vi "SMS_to_mobile.vi"(1 "SMS address":string[](array[string])=["SMS to Mobile:enflo@froude.mech.surrey.ac.uk"], 2 "Subject":string="Comms check", 3 "Message":string) -> (5 "error out":errorcluster)   [LabVIEW 2010]
uses:
  Globals/Preference_global.vi
panel:
  in  "Case Constant\n(See Context Help)":bool
  out "Number of SMS's sent today":i32
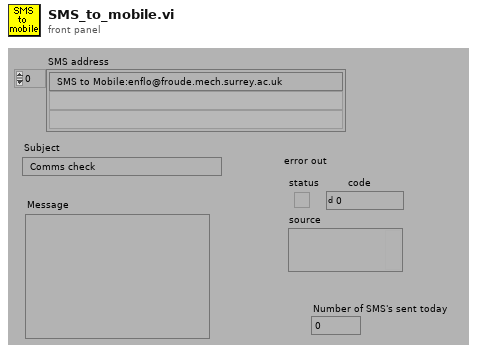
[diagram p1: front panel]
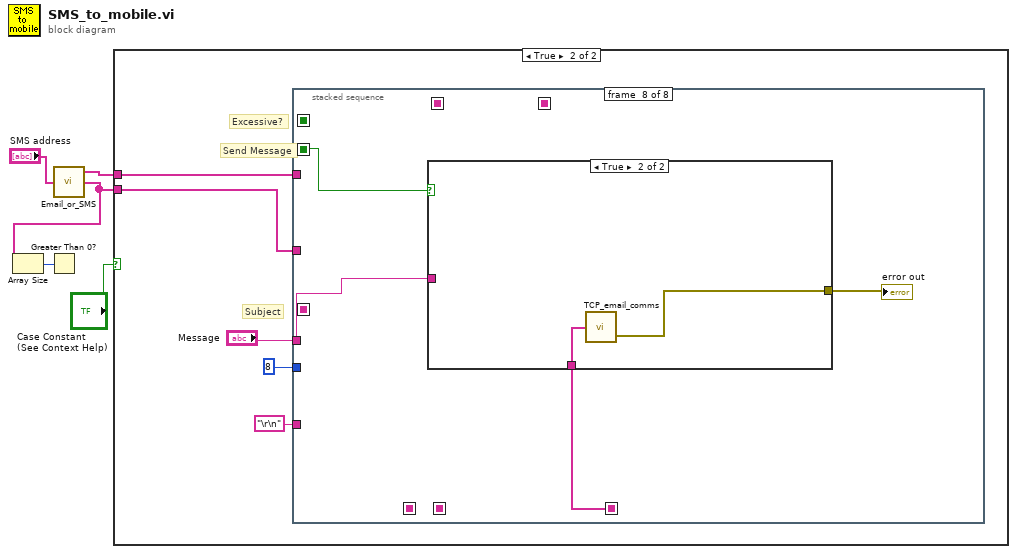
[diagram p0: block diagram]
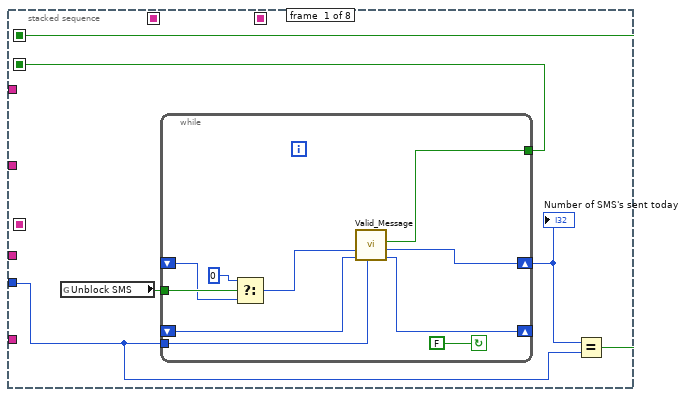
[diagram p3: hidden frame]
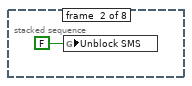
[diagram p4: hidden frame]
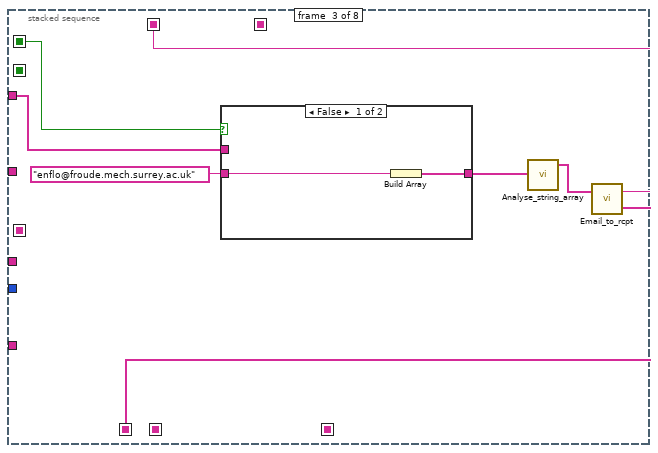
[diagram p5: hidden frame]
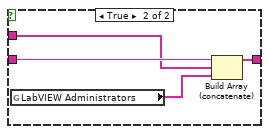
[diagram p6: hidden frame]
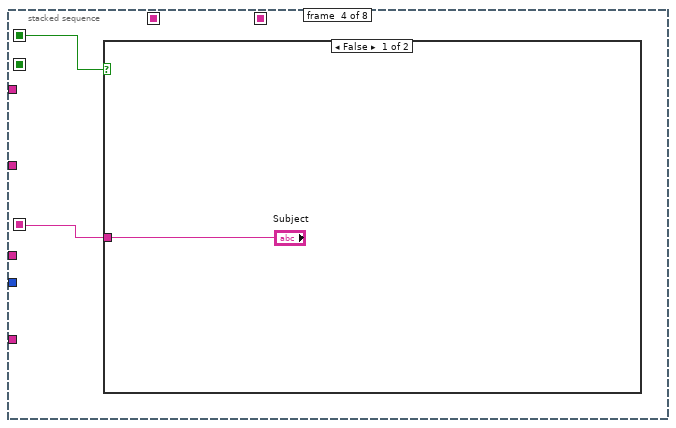
[diagram p7: hidden frame]
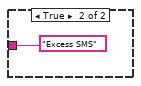
[diagram p8: hidden frame]
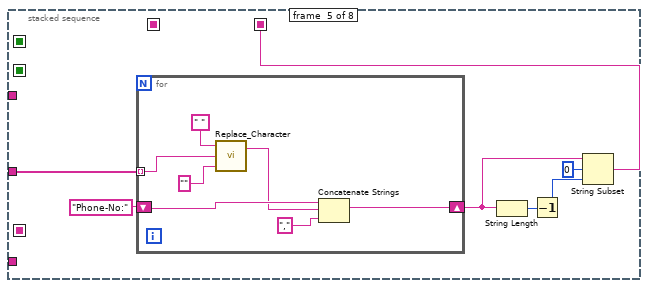
[diagram p9: hidden frame]
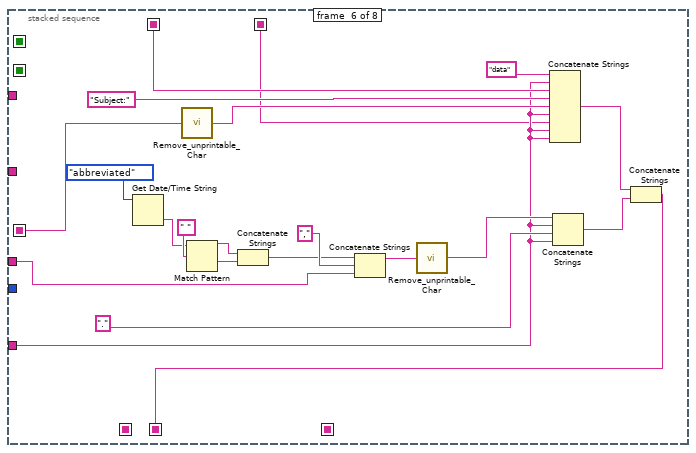
[diagram p10: hidden frame]
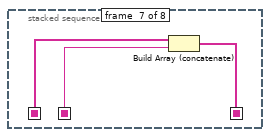
[diagram p11: hidden frame]
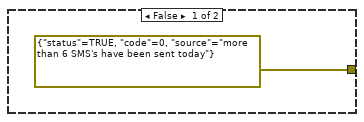
[diagram p12: hidden frame]
diagram:
  n1 = call "Email_or_SMS.vi"("Email address"="SMS address") -> ("Email"=w3:string[], "SMS to send"=w2:string[])  [unwired: 2 out]
  n2 = Array Size(array=w2) -> (size(s)=w4:i32)
  n3 = Greater Than 0?(x=w4) -> ()  [unwired: 1 out]
  n4 = case shown="True" "Case Constant\n(See Context Help)" {
    tunnel: w2 -> [_ w6]
    tunnel: w3 -> [_ w7]
    frame False {
    }
    frame True {
      # "Subject"
      # "Send Message"
      # "Excessive?"
      n5 = stacked-sequence {
        seq-local: [_ _ w28 _ _ _ _ _] -> [_ _ _ _ _ _ w80 _]
        seq-local: [_ _ w29 _ _ _ _ _] -> [_ _ _ _ _ w77 _ _]
        seq-local: [_ _ _ _ _ w73 _ _] -> [_ _ _ _ _ _ w81 _]
        seq-local: [_ _ _ _ _ _ w79 _] -> [_ _ _ _ _ _ _ w83]
        seq-local: [w14 _ _ _ _ _ _ _] -> [_ _ _ _ _ _ _ w84]
        seq-local: [w11 _ _ _ _ _ _ _] -> [_ _ w33 w40 _ _ _ _]
        seq-local: [_ _ _ w41 _ _ _ _] -> [_ _ _ _ _ w61 _ _]
        seq-local: [_ _ _ _ w44 _ _ _] -> [_ _ _ _ _ w58 _ _]
        tunnel: "\r\n" -> [_ _ _ _ _ w59 _ _]
        tunnel: w6 -> [_ _ _ _ w50 _ _ _]
        tunnel: 8 ("y") -> [w13 _ _ _ _ _ _ _]
        tunnel: "Message" -> [_ _ _ _ _ w60 _ w82]
        tunnel: w7 -> [_ _ w32 _ _ _ _ _]
        frame #0 {
          n6 = global read "Preference_global.vi" "Unblock SMS"() -> (w15:bool)
          n7 = while {
            tunnel: w15 -> [w20]
            tunnel: w13 -> [w22]
            tunnel: [w23] -> w14
            shift-left: _ -> [w19]
            shift-right: [w21] -> w12
            shift-left: _ -> [w25]
            shift-right: [w24] -> _
            stop <- FALSE continue-if-true
            n8 = Select(t=0, s=w20, f=w19) -> (s? t:f=w18:i32)
            n9 = call "Valid_Message.vi"("Max per day"=w22, "day of month in"=w25, "Number of requests today In"=w18) -> ("day of month out"=w24:i32, "Number of requests today Out"=w21:i32, "Send Message"=w23:bool)  [unwired: 2 in, 4 out]
          }
          "Number of SMS's sent today" <- w12
          n10 = Equal?(x=w12, y=w13) -> (x = y?=w11:bool)
        }
        frame #1 {
          n11 = global write "Preference_global.vi" "Unblock SMS"(FALSE ("Unblock Email")) -> ()
        }
        frame #2 {
          n12 = case shown="False" w33 {
            tunnel: "enflo@froude.mech.surrey.ac.uk" -> [w35 w38]
            tunnel: [w34 w39] -> w31
            tunnel: w32 -> [_ w37]
            frame False {
              n13 = Build Array(w35) -> (w34:string[])
            }
            frame True {
              n14 = global read "Preference_global.vi" "LabVIEW Administrators"() -> (w36:string[])
              n15 = Build Array (concatenate)(w38, w37, w36) -> (w39:string[])
            }
          }
          n16 = call "Analyse_string_array.vi"("String array"=w31) -> ("Unique strings"=w30:string[])  [unwired: 2 out]
          n17 = call "Email_to_rcpt.vi"("Email Addresses"=w30) -> ("rcpt to"=w28:string[], "To"=w29:string)  [unwired: 1 out]
        }
        frame #3 {
          n18 = case shown="False" w40 {
            tunnel: ["Subject" "Excess SMS" ("Email address")] -> w41
            frame False {
            }
            frame True {
            }
          }
        }
        frame #4 {
          n19 = for {
            shift-right: [w55] -> w45
            shift-left: "Phone-No:" -> [w57]
            tunnel: w50 -> [w52] mode=indexing
            n20 = call "Replace_Character.vi"("Replace with"="", "Input String"=w52, "Search For"=" ") -> ("Output string"=w51:string)  [unwired: 1 out]
            n21 = Concatenate Strings(w57, w51, "," ("Substring")) -> (w55:string)
          }
          n22 = String Length(string=w45) -> (length=w47:i32)
          n23 = Decrement(x=w47) -> (x-1=w46:i32)
          n24 = String Subset(string=w45, offset (0)=0, length (rest)=w46) -> (substring=w44:string)
        }
        frame #5 {
          n25 = Get Date/Time String(date format (0)=enum16{"short", "long", "abbreviated"}."abbreviated") -> (time string=w65:string)  [unwired: 3 out]
          n26 = call "Remove_unprintable_Char.vi"("Input String"=w61) -> ("Output String"=w71:string)
          n27 = Match Pattern(string=w65, regular expression=" ") -> (before substring=w69:string, after substring=w70:string)  [unwired: 3 out]
          n28 = Concatenate Strings(w69, w70) -> (w64:string)
          n29 = Concatenate Strings(w64, "," ("regular expression"), w60) -> (w63:string)
          n30 = call "Remove_unprintable_Char.vi"("Input String"=w63) -> ("Output String"=w62:string)
          n31 = Concatenate Strings("data", w59, w77, "Subject:", w71, w59, w58, w59, w59) -> (w75:string)
          n32 = Concatenate Strings(w62, w59, ".", w59) -> (w74:string)
          n33 = Concatenate Strings(w75, w74) -> (w73:string)
        }
        frame #6 {
          n34 = Build Array (concatenate)(w80, w81) -> (w79:string[])
        }
        frame #7 {
          n35 = case shown="True" w84 {
            tunnel: [errorcluster {"status"=TRUE, "code"=0, "source"="more than 6 SMS's have been sent today"} ("error out") w88] -> w85
            tunnel: w83 -> [_ w87]
            tunnel: w82 -> [_ _]
            frame False {
            }
            frame True {
              n36 = call "TCP_email_comms.vi"("Commands Array"=w87) -> ("error out"=w88:errorcluster)  [unwired: 1 out]
            }
          }
          "error out" <- w85
        }
      }
    }
  }
